vi "GUI alphanumeric + dash character filter.vi"(1 "Char":i16) -> (0 "Discard?":bool)   [LabVIEW 2012, in "Strings Lib.lvlib"]
uses:
  Strings Lib.lvlib
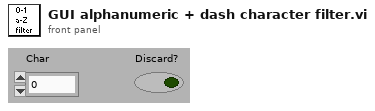
[diagram p1: front panel]
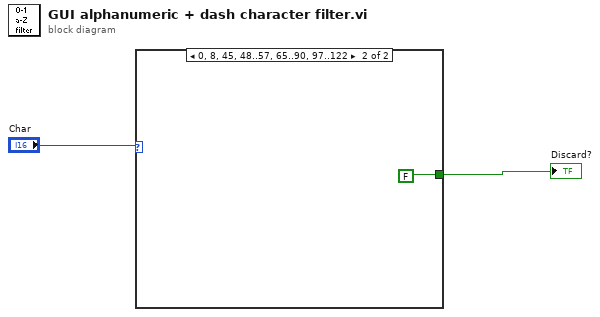
[diagram p0: block diagram]
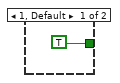
[diagram p2: hidden frame]
diagram:
  n1 = case shown="0, 8, 45, 48..57, 65..90, 97..122" "Char" {
    tunnel: [TRUE FALSE] -> w2
    frame 1, Default {
    }
    frame 0, 8, 45, 48..57, 65..90, 97..122 {
    }
  }
  "Discard?" <- w2
